vi "Add-log-message-action.vi"(8 "error in (no error)":errorcluster, 9 "Motor index":i32, 10 "Action":refnum<class "Action.lvclass">, 11 "Activity log":refnum<user-event>) -> (0 "error out":errorcluster, 3 "Activity log dup":refnum<user-event>)   [LabVIEW 2013, in "PowderDeposition.lvlib" / "PD-Main.lvclass"]
uses:
  PD-Main.lvclass
  Action/Action.lvclass
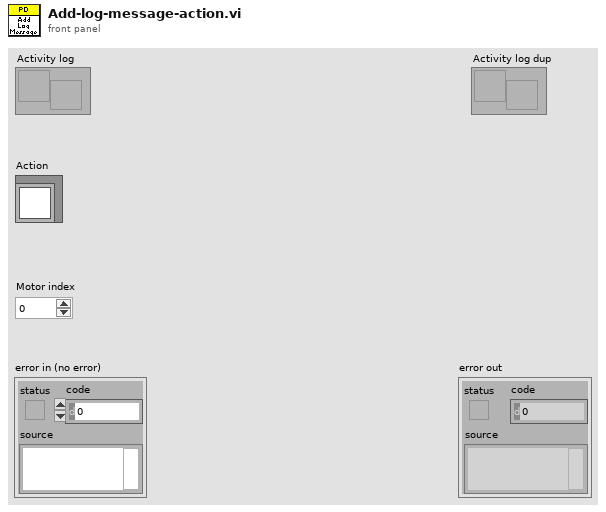
[diagram p1: front panel]
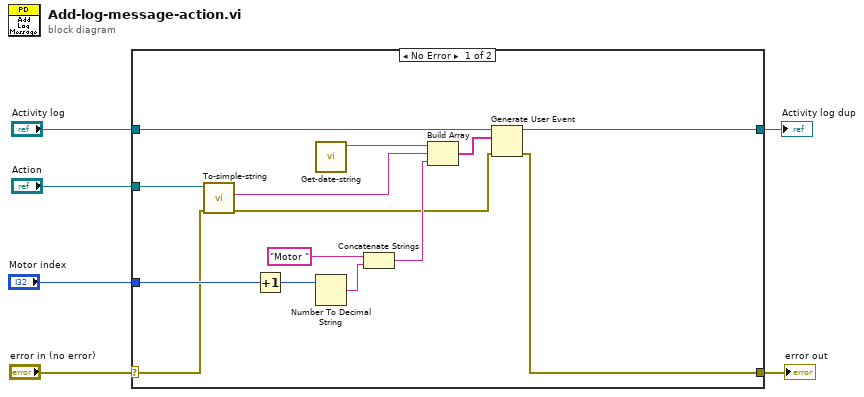
[diagram p0: block diagram]
diagram:
  n1 = case shown="No Error" "error in (no error)" {
    selector: "error in (no error)" -> [w9 w22]
    tunnel: [w14 w22] -> w5
    tunnel: "Action" -> [w10 _]
    tunnel: "Motor index" -> [w19 _]
    tunnel: "Activity log" -> [w12 w21]
    tunnel: [w11 w21] -> w2
    frame No Error {
      n2 = call-dynamic "To-simple-string.vi"("error in (no error)"=w9, "Action in"=w10) -> ("error out"=w8:errorcluster, "Action string"=w7:string)  [unwired: 7 in, 1 out]
      n3 = Increment(x=w19) -> (x+1=w13:i32)
      n4 = call "Get-date-string.vi"() -> ("Date string"=w20:string)  [unwired: 11 in]
      n5 = Number To Decimal String(number=w13) -> (decimal integer string=w18:string)  [unwired: 1 in]
      n6 = Concatenate Strings("Motor ", w18) -> (w16:string)
      n7 = Build Array(w20, w7, w16) -> (w15:string[])
      n8 = Generate User Event(user event=w12, event data cluster=w15, error in=w8) -> (user event out=w11:refnum<user-event>, error out=w14:errorcluster)  [unwired: 1 in]
    }
    frame Error {
    }
  }
  "error out" <- w5
  "Activity log dup" <- w2
